vi "Raw List String.vi"(8 "error in (no error)":errorcluster, 10 "Remote File":string, 11 "FTP in":refnum<class "FTP.lvclass">) -> (0 "error out":errorcluster, 2 "Raw List as String":string, 3 "FTP out":refnum<class "FTP.lvclass">)   [LabVIEW 2013, in "FTP.lvlib" / "FTP.lvclass"]
uses:
  FTP.lvclass
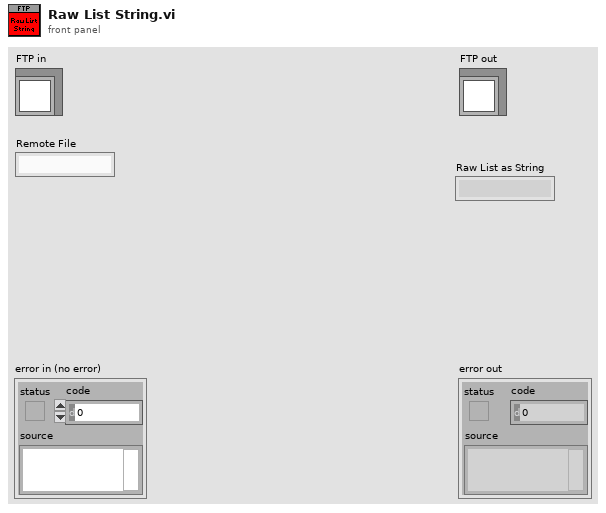
[diagram p1: front panel]
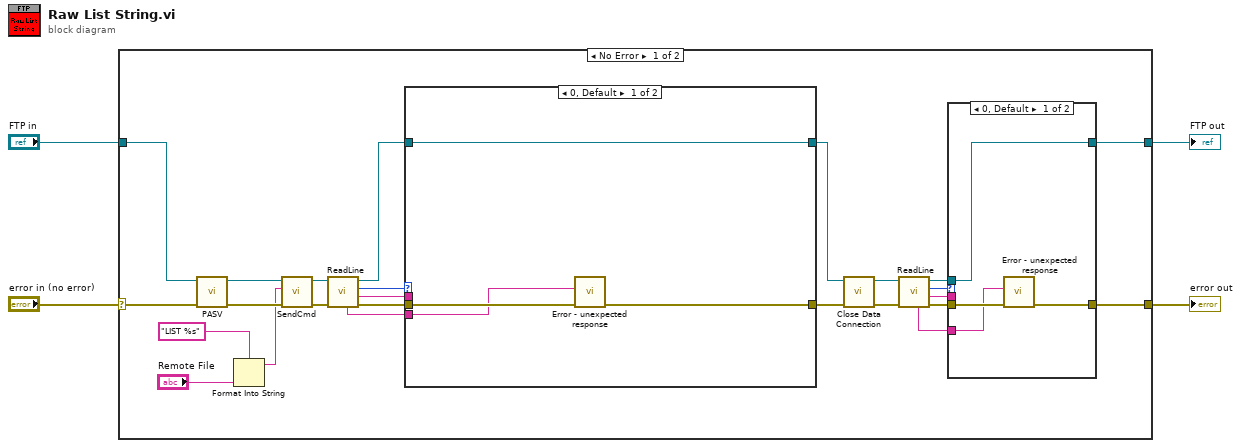
[diagram p0: block diagram]
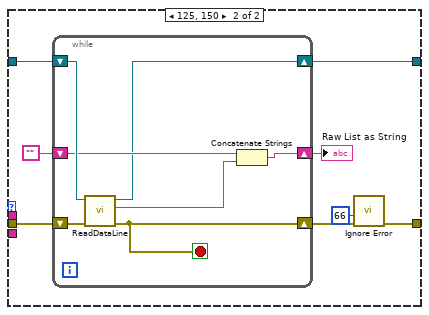
[diagram p3: hidden frame]
diagram:
  n1 = case shown="No Error" "error in (no error)" {
    selector: "error in (no error)" -> [w7 w56]
    tunnel: [w9 w56] -> w3
    tunnel: [w10 w55] -> w1
    tunnel: "FTP in" -> [w8 w55]
    frame No Error {
      n2 = call "PASV.vi"("error in (no error)"=w7, "FTP in"=w8) -> ("error out"=w26:errorcluster, "FTP out"=w27:refnum<class "FTP.lvclass">)  [unwired: 8 in]
      n3 = Format Into String(format string="LIST %s" ("cmd"), "Remote File") -> (resulting string=w11:string)  [unwired: 2 in, 1 out]
      n4 = call "SendCmd.vi"("error in (no error)"=w26, "cmd"=w11, "FTP in"=w27) -> ("error out"=w28:errorcluster, "FTP out"=w29:refnum<class "FTP.lvclass">)  [unwired: 7 in]
      n5 = call "ReadLine.vi"("error in (no error)"=w28, "FTP in"=w29) -> ("error out"=w25:errorcluster, "Line"=w23:string, "code"=w24:i32, "FTP out"=w22:refnum<class "FTP.lvclass">, "Full Line"=w5:string)  [unwired: 5 in]
      n6 = case shown="0, Default" w24 {
        tunnel: w25 -> [w38 w47]
        tunnel: w22 -> [w39 w46]
        tunnel: [w36 w43] -> w15
        tunnel: [w39 w45] -> w14
        tunnel: w23 -> [_ _]
        tunnel: w5 -> [w37 _]
        frame 0, Default {
          n7 = call "Error - unexpected response.vi"("error in (no error)"=w38, "Full Response"=w37) -> ("error out"=w36:errorcluster)  [unwired: 9 in]
        }
        frame 125, 150 {
          n8 = while {
            shift-right: [w49] -> w44
            shift-left: w47 -> [w54]
            shift-right: [w48] -> w45
            shift-left: w46 -> [w53]
            shift-right: [w52] -> w40
            shift-left: "" -> [w51]
            stop <- w49 stop-if-true
            n9 = call "ReadDataLine.vi"("error in (no error)"=w54, "FTP in"=w53) -> ("error out"=w49:errorcluster, "Data"=w50:string, "FTP out"=w48:refnum<class "FTP.lvclass">)  [unwired: 7 in]
            n10 = Concatenate Strings(w51, w50) -> (w52:string)
          }
          "Raw List as String" <- w40
          n11 = call "Ignore Error.vi"("error in"=w44, "code"=66) -> ("error out"=w43:errorcluster)  [unwired: 9 in]
        }
      }
      n12 = call "Close Data Connection.vi"("error in (no error)"=w15, "FTP in"=w14) -> ("error out"=w21:errorcluster, "FTP out"=w20:refnum<class "FTP.lvclass">)  [unwired: 8 in]
      n13 = call "ReadLine.vi"("error in (no error)"=w21, "FTP in"=w20) -> ("error out"=w19:errorcluster, "Line"=w16:string, "code"=w18:i32, "FTP out"=w17:refnum<class "FTP.lvclass">, "Full Line"=w6:string)  [unwired: 5 in]
      n14 = case shown="0, Default" w18 {
        tunnel: w19 -> [w32 w34]
        tunnel: [w31 w34] -> w9
        tunnel: w17 -> [w33 w35]
        tunnel: [w33 w35] -> w10
        tunnel: w16 -> [_ _]
        tunnel: w6 -> [w30 _]
        frame 0, Default {
          n15 = call "Error - unexpected response.vi"("error in (no error)"=w32, "Full Response"=w30) -> ("error out"=w31:errorcluster)  [unwired: 9 in]
        }
        frame 226 {
        }
      }
    }
    frame Error {
    }
  }
  "error out" <- w3
  "FTP out" <- w1
